vi "Update Slaved Digital.vi"(8 "error in (no error)":errorcluster, 9 "Output States":bool[](array[boolean]), 10 "Master Channel Number":i32, 11 "Master Device in":refnum<class "Master Device.lvclass">) -> (0 "error out":errorcluster, 3 "Master Device out":refnum<class "Master Device.lvclass">)   [LabVIEW 2013, in "Master Device.lvclass"]
uses:
  Master Device.lvclass
  Master Device.lvclass/Master Device.ctl
  <vilib>/Utility/error.llb/DialogType.ctl
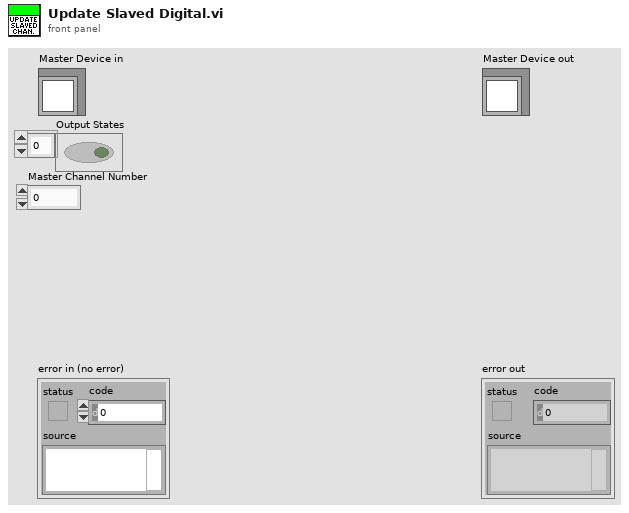
[diagram p1: front panel]
types:
  T1 = cluster{"Master Channel Number":i32, "Output States":bool[]}
  T2 = cluster{"Master Channel Number":i32, "Output States":bool[]}[]
  T3 = typedef "DialogType.ctl" = u16
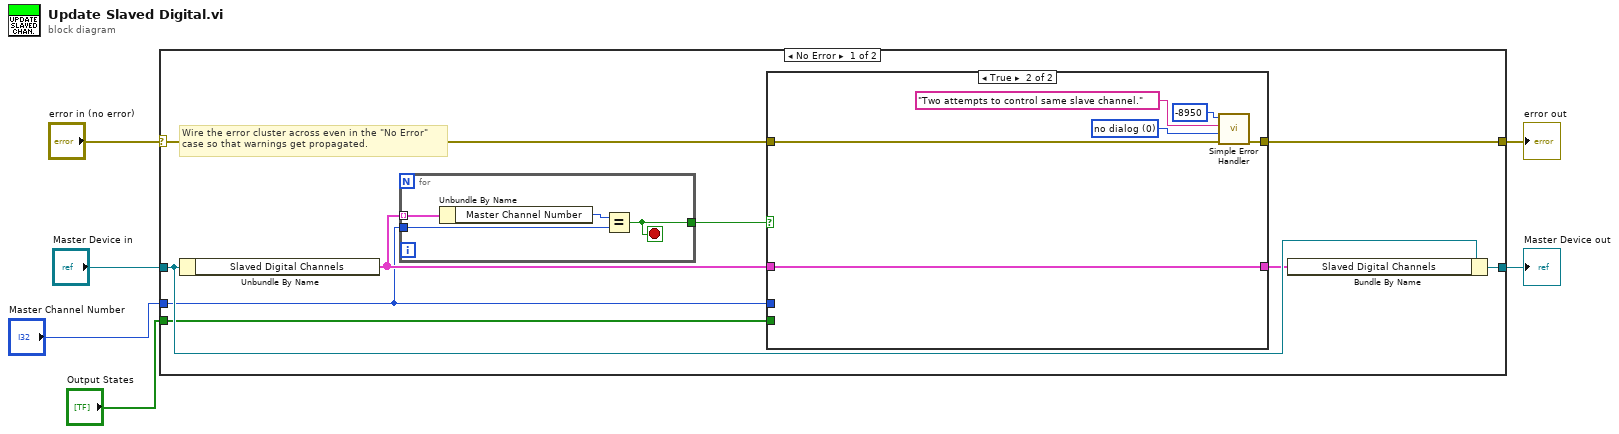
[diagram p0: block diagram]
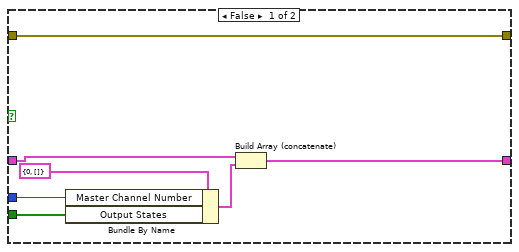
[diagram p2: hidden frame]
diagram:
  n1 = case shown="No Error" "error in (no error)" {
    selector: "error in (no error)" -> [w9 w34]
    tunnel: [w8 w34] -> w5
    tunnel: [w15 w33] -> w3
    tunnel: "Master Device in" -> [w14 w33]
    tunnel: "Master Channel Number" -> [w10 _]
    tunnel: "Output States" -> [w12 _]
    frame No Error {
      # "Wire the error cluster across even in the \"No Error\"\ncase so that warnings get propagated."
      n2 = Unbundle By Name(w14) -> ("Slaved Digital Channels"=w11:T2)
      n3 = for {
        tunnel: w11 -> [w32] mode=indexing
        tunnel: w10 -> [w31]
        tunnel: [w29] -> w7
        stop <- w29 stop-if-true
        n4 = Unbundle By Name(w32) -> ("Master Channel Number"=w30:i32)
        n5 = Equal?(x=w30, y=w31) -> (x = y?=w29:bool)
      }
      n6 = case shown="True" w7 {
        tunnel: [w21 w28] -> w13
        tunnel: w12 -> [w19 _]
        tunnel: w11 -> [w18 w28]
        tunnel: w10 -> [w17 _]
        tunnel: w9 -> [w16 w26]
        tunnel: [w16 w27] -> w8
        frame False {
          n7 = Bundle By Name(cluster=T1 {"Master Channel Number"=0, "Output States"=[]} ("Slaved Digital Channel"), "Master Channel Number"=w17, "Output States"=w19) -> (w20:T1)
          n8 = Build Array (concatenate)(w18, w20) -> (w21:T2)
        }
        frame True {
          w23 = T3 0 items=["no dialog", "OK message", "continue or stop message", "OK message + warnings", "continue/stop + warnings"] ("type of dialog (OK msg:1)")
          n9 = call <vilib>:"Simple Error Handler.vi"("error code (no error:0)"=-8950, "error source (\" \")"="Two attempts to control same slave channel." ("error source (\" \")"), "type of dialog (OK msg:1)"=w23, "error in (no error)"=w26) -> ("error out"=w27:errorcluster)  [unwired: 1 in, 4 out]
        }
      }
      n10 = Bundle By Name(cluster=w14, "Slaved Digital Channels"=w13) -> (w15:refnum<class "Master Device.lvclass">)
    }
    frame Error {
    }
  }
  "error out" <- w5
  "Master Device out" <- w3
